vi "read default value Double.vi"(8 "error in":errorcluster, 11 "system tag in":refnum<class "data bus tag description.lvclass">) -> (0 "error out":errorcluster, 1 "invalid":bool, 2 "default value":dbl, 3 "system tag out":refnum<class "data bus tag description.lvclass">)   [LabVIEW 2013, in "data bus tag description.lvclass"]
doc: "Converts the raw default value stored in the tag to the type specified by the polymorph."
uses:
  data bus tag description.lvclass
  Data Type.ctl
  data bus tag description.lvclass/data bus tag description.ctl
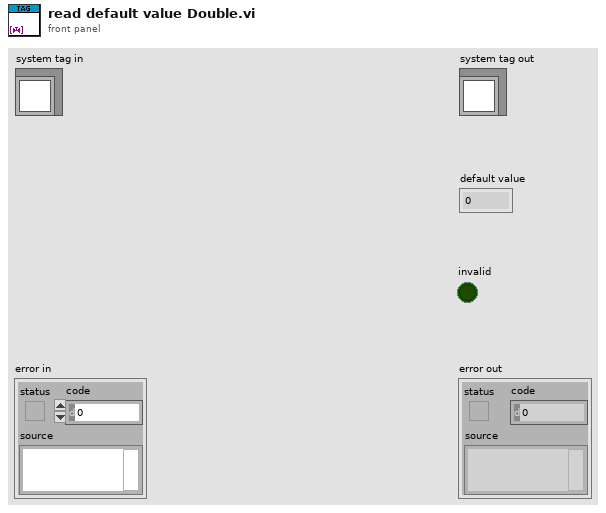
[diagram p1: front panel]
types:
  T1 = typedef "data bus tag description.lvclass/Data Type.ctl" = enum16{"Double", "I64", "Boolean", "Array of Double", "Array of I64", "Variant"}
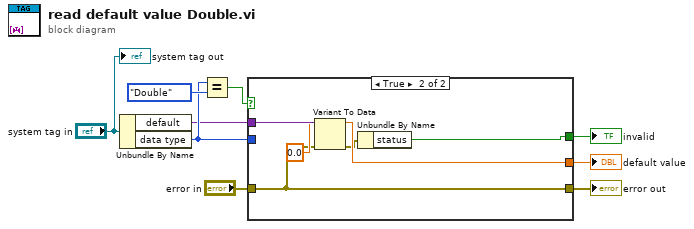
[diagram p0: block diagram]
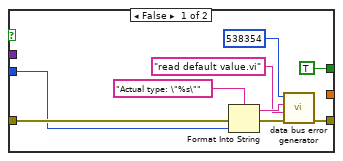
[diagram p2: hidden frame]
diagram:
  n1 = Unbundle By Name("system tag in") -> ("default"=w3:variant, "data type"=w4:T1)
  n2 = Equal?(x=w4, y=Data_Type."Double") -> (x = y?=w7:bool)
  n3 = case shown="True" w7 {
    tunnel: "error in" -> [w18 w22]
    tunnel: [w14 w22] -> w5
    tunnel: w4 -> [w13 _]
    tunnel: w3 -> [_ w24]
    tunnel: [_ w21] -> w2
    tunnel: [TRUE ("status") w19] -> w1
    frame False {
      n4 = Format Into String(format string="Actual type: \"%s\"", error in=w18, w13) -> (resulting string=w15:string, error out=w16:errorcluster)  [unwired: 1 in]
      n5 = call "data bus error generator.vi"("error in"=w16, "source"="read default value.vi", "append error message"=w15, "error code (0)"=538354) -> ("error out"=w14:errorcluster)  [unwired: 5 in]
    }
    frame True {
      n6 = Variant To Data(error in=w22, type=0.0 ("default value 1"), Variant=w24) -> (data=w21:dbl, error out=w20:errorcluster)
      n7 = Unbundle By Name(w20) -> ("status"=w19:bool)
    }
  }
  "error out" <- w5
  "default value" <- w2
  "invalid" <- w1
  "system tag out" <- "system tag in"
